vi "Get Gradient Threshold.vi"(8 "error in (no error)":errorcluster, 11 "Barcode Detector in":refnum<class "Barcode Detector.lvclass">) -> (0 "error out":errorcluster, 2 "Threshold":dbl, 3 "Barcode Detector (Duplicate)":refnum<class "Barcode Detector.lvclass">)   [LabVIEW 2020, in "feature_detection.lvlib" / "Barcode Detector.lvclass"]
uses:
  Barcode Detector.lvclass
  Barcode Detector.lvclass/Barcode Detector.ctl
  common/Module Path.vi
  <vilib>/Utility/error.llb/Error Cluster From Error Code.vi
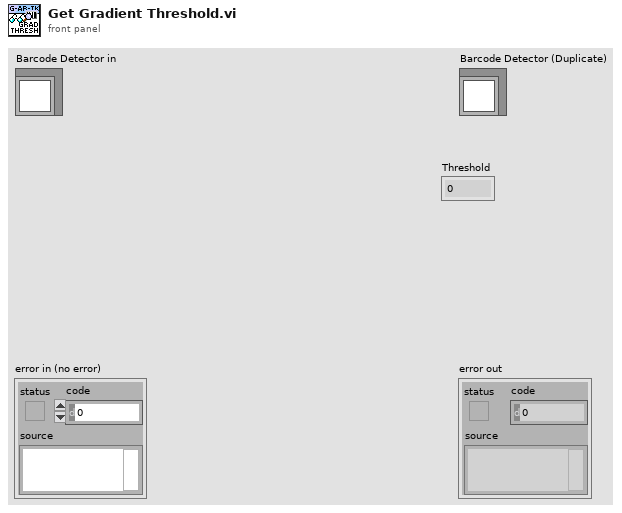
[diagram p1: front panel]
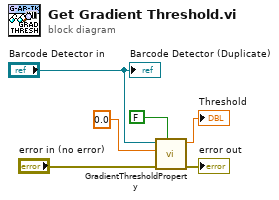
[diagram p0: block diagram]
diagram:
  n1 = call "GradientThresholdProperty.vi"("Write?"=FALSE, "error in (no error)"="error in (no error)", "Value in"=0.0 ("Value"), "Barcode Detector in"="Barcode Detector in") -> ("error out"=→"error out":errorcluster, "Value out"=→"Threshold":dbl)  [unwired: 6 in]
  "Barcode Detector (Duplicate)" <- "Barcode Detector in"
